vi "Read SequesDone.vi"(8 "error in (no error)":errorcluster, 11 "Channel in":refnum<class "Channel.lvclass">) -> (0 "error out":errorcluster, 1 "SequesDoneRaw":u32, 2 "SequesDone":u32, 3 "Channel out":refnum<class "Channel.lvclass">)   [LabVIEW 2018, in "Channel.lvclass"]
uses:
  Channel.lvclass
  Channel.lvclass/Channel.ctl
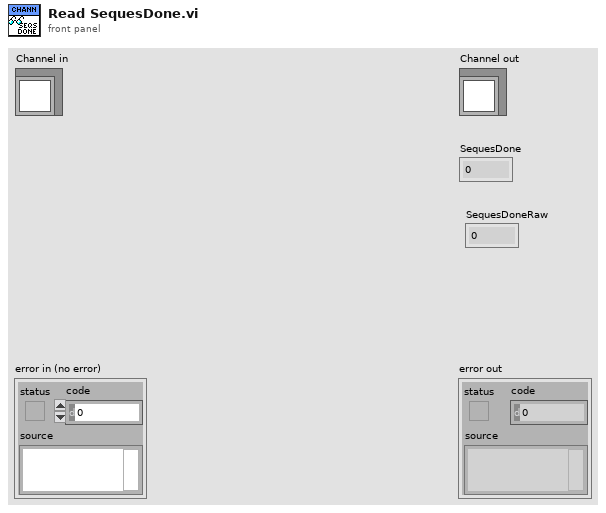
[diagram p1: front panel]
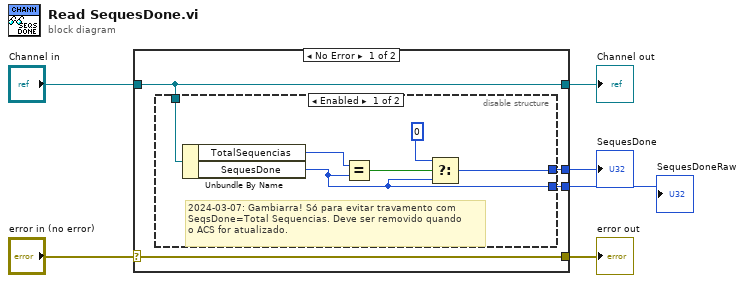
[diagram p0: block diagram]
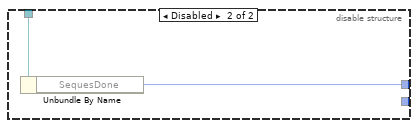
[diagram p2: hidden frame]
diagram:
  n1 = case shown="No Error" "error in (no error)" {
    selector: "error in (no error)" -> [w10 w19]
    tunnel: [w10 w19] -> w5
    tunnel: [w9 w20] -> w3
    tunnel: "Channel in" -> [w9 w20]
    tunnel: [w8 _] -> w2
    tunnel: [w7 _] -> w1
    frame No Error {
      n2 = disable-structure shown="Enabled" {
        disable-tunnel: w9 -> [w16 w18]
        disable-tunnel: [w15 w17] -> w8
        disable-tunnel: [w11 _] -> w7
        frame Enabled {
          # "2024-03-07: Gambiarra! Só para evitar travamento com\nSeqsDone=Total Sequencias. Deve ser removido quando\no ACS for atualizado."
          n3 = Unbundle By Name(w16) -> ("TotalSequencias"=w13:u32, "SequesDone"=w11:u32)
          n4 = Equal?(x=w13, y=w11) -> (x = y?=w14:bool)
          n5 = Select(t=0, s=w14, f=w11) -> (s? t:f=w15:u32)
        }
        frame Disabled {
          n6 = Unbundle By Name(w18) -> ("SequesDone"=w17:u32)
        }
      }
    }
    frame Error {
    }
  }
  "error out" <- w5
  "Channel out" <- w3
  "SequesDone" <- w2
  "SequesDoneRaw" <- w1
